vi "Get cif_manager_PluginInfo.vi"(8 "error in (no error)":errorcluster, 11 "gRPCid":T1) -> (0 "error out":errorcluster, 2 "package_templatemessage":T2, 3 "gRPCid out":T1)   [LabVIEW 2021, in "CIF_Launcher_server.lvlib"]
uses:
  CIF_Launcher_server.lvlib
  cif_manager_PluginInfo.ctl
  cif_common_ShortVersion.ctl
  cif_plugincore_StatusData.ctl
  cif_plugincore_StatusData_PluginState.ctl
  cif_plugincore_TimingStatistics.ctl
  cif_common_TimingStats.ctl
  cif_plugincore_FifoStatistics.ctl
  cif_plugincore_Error.ctl
  cif_plugincore_MonitorDoubles.ctl
  cif_plugincore_MonitorU64.ctl
  cif_plugincore_MonitorI64.ctl
  <vilib>/gRPC/LabVIEW gRPC Library/Shared/grpcId.ctl
  cif_manager_PluginInfo_Flat.ctl
  cif_common_ShortVersion_Flat.ctl
  cif_plugincore_StatusData_Flat.ctl
  cif_plugincore_TimingStatistics_Flat.ctl
  cif_common_TimingStats_Flat.ctl
  cif_plugincore_FifoStatistics_Flat.ctl
  cif_plugincore_Error_Flat.ctl
  cif_plugincore_MonitorDoubles_Flat.ctl
  cif_plugincore_MonitorU64_Flat.ctl
  cif_plugincore_MonitorI64_Flat.ctl
  2ed25e12-861d-4677-8ead-ace2906b2041.vi
  <vilib>/gRPC/LabVIEW gRPC Library/Shared/TranslateGrpcError.vi
  FlatToRichcif_common_ShortVersion.vi
  FlatToRichcif_plugincore_StatusData.vi
  FlatToRichcif_plugincore_TimingStatistics.vi
  FlatToRichcif_plugincore_FifoStatistics.vi
  FlatToRichcif_plugincore_Error.vi
  FlatToRichcif_plugincore_MonitorDoubles.vi
  FlatToRichcif_plugincore_MonitorU64.vi
  FlatToRichcif_plugincore_MonitorI64.vi
  FlatToRichcif_common_TimingStats.vi
  <vilib>/gRPC/LabVIEW gRPC Library/Server API/Server/Get Server DLL Path.vi
  <vilib>/Utility/error.llb/Error Cluster From Error Code.vi
  <vilib>/gRPC/LabVIEW gRPC Library/grpc-lvsupport-release.lvlib
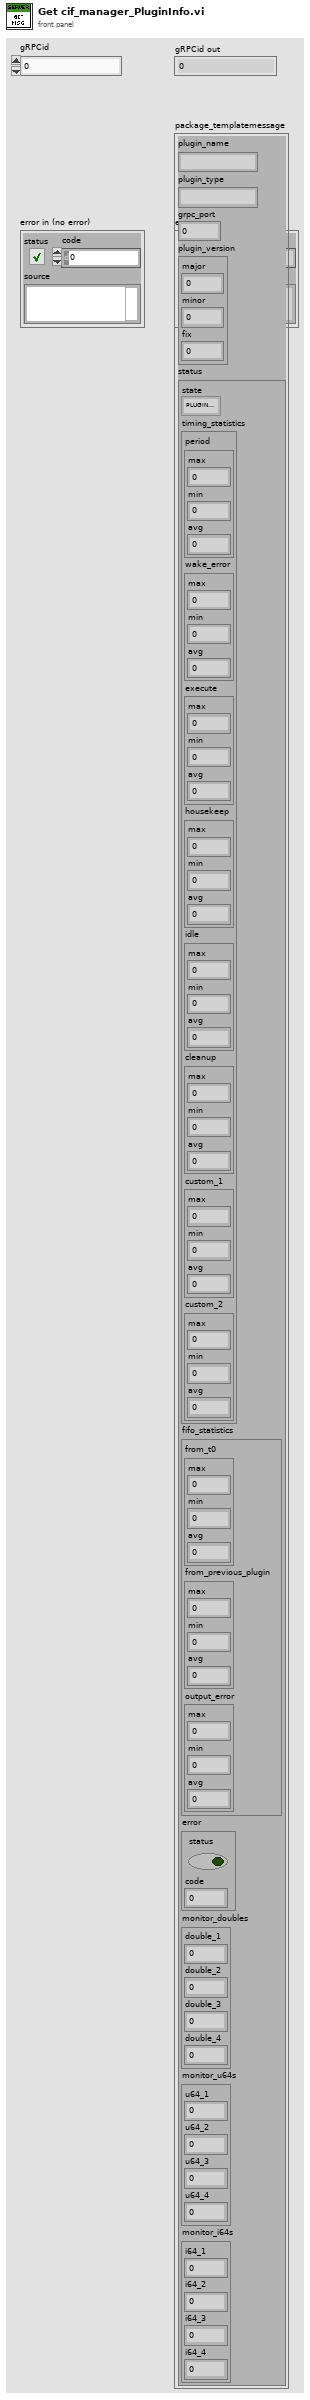
[diagram p1: front panel]
types:
  T1 = typedef "grpc-lvsupport-release.lvlib/grpcId.ctl" = u64
  T2 = typedef "CIF_Launcher_server.lvlib/cif_manager_PluginInfo.ctl" = cluster{"plugin_name":string, "plugin_type":string, "grpc_port":i32, "plugin_version":T3, "status":T4}
  T3 = typedef "CIF_Launcher_server.lvlib/cif_common_ShortVersion.ctl" = cluster{"major":u32, "minor":u32, "fix":u32}
  T4 = typedef "CIF_Launcher_server.lvlib/cif_plugincore_StatusData.ctl" = cluster{"state":T5, "timing_statistics":T6, "fifo_statistics":T8, "error":T9, "monitor_doubles":T10, "monitor_u64s":T11, "monitor_i64s":T12}
  T5 = typedef "CIF_Launcher_server.lvlib/cif_plugincore_StatusData_PluginState.ctl" = enum32{"PLUGINSTATE_UNKNOWN", "PLUGINSTATE_CREATING", "PLUGINSTATE_LISTENING", "PLUGINSTATE_RUNNING", "PLUGINSTATE_CLEANINGUP", "PLUGINSTATE_DESTROYING"}
  T6 = typedef "CIF_Launcher_server.lvlib/cif_plugincore_TimingStatistics.ctl" = cluster{"period":T7, "wake_error":T7, "execute":T7, "housekeep":T7, "idle":T7, "cleanup":T7, "custom_1":T7, "custom_2":T7}
  T7 = typedef "CIF_Launcher_server.lvlib/cif_common_TimingStats.ctl" = cluster{"max":i64, "min":i64, "avg":dbl}
  T8 = typedef "CIF_Launcher_server.lvlib/cif_plugincore_FifoStatistics.ctl" = cluster{"from_t0":T7, "from_previous_plugin":T7, "output_error":T7}
  T9 = typedef "CIF_Launcher_server.lvlib/cif_plugincore_Error.ctl" = cluster{"status":bool, "code":i32}
  T10 = typedef "CIF_Launcher_server.lvlib/cif_plugincore_MonitorDoubles.ctl" = cluster{"double_1":dbl, "double_2":dbl, "double_3":dbl, "double_4":dbl}
  T11 = typedef "CIF_Launcher_server.lvlib/cif_plugincore_MonitorU64.ctl" = cluster{"u64_1":u64, "u64_2":u64, "u64_3":u64, "u64_4":u64}
  T12 = typedef "CIF_Launcher_server.lvlib/cif_plugincore_MonitorI64.ctl" = cluster{"i64_1":i64, "i64_2":i64, "i64_3":i64, "i64_4":i64}
  T13 = typedef "CIF_Launcher_server.lvlib/cif_manager_PluginInfo_Flat.ctl" = cluster{"plugin_name":string, "plugin_type":string, "grpc_port":i32, "plugin_version":T14, "status":T15}
  T14 = typedef "CIF_Launcher_server.lvlib/cif_common_ShortVersion_Flat.ctl" = cluster{"major":u32, "minor":u32, "fix":u32}
  T15 = typedef "CIF_Launcher_server.lvlib/cif_plugincore_StatusData_Flat.ctl" = cluster{"state":T5, "timing_statistics":T16, "fifo_statistics":T18, "error":T19, "monitor_doubles":T20, "monitor_u64s":T21, "monitor_i64s":T22}
  T16 = typedef "CIF_Launcher_server.lvlib/cif_plugincore_TimingStatistics_Flat.ctl" = cluster{"period":T17, "wake_error":T17, "execute":T17, "housekeep":T17, "idle":T17, "cleanup":T17, "custom_1":T17, "custom_2":T17}
  T17 = typedef "CIF_Launcher_server.lvlib/cif_common_TimingStats_Flat.ctl" = cluster{"max":i64, "min":i64, "avg":dbl}
  T18 = typedef "CIF_Launcher_server.lvlib/cif_plugincore_FifoStatistics_Flat.ctl" = cluster{"from_t0":T17, "from_previous_plugin":T17, "output_error":T17}
  T19 = typedef "CIF_Launcher_server.lvlib/cif_plugincore_Error_Flat.ctl" = cluster{"status":bool, "code":i32}
  T20 = typedef "CIF_Launcher_server.lvlib/cif_plugincore_MonitorDoubles_Flat.ctl" = cluster{"double_1":dbl, "double_2":dbl, "double_3":dbl, "double_4":dbl}
  T21 = typedef "CIF_Launcher_server.lvlib/cif_plugincore_MonitorU64_Flat.ctl" = cluster{"u64_1":u64, "u64_2":u64, "u64_3":u64, "u64_4":u64}
  T22 = typedef "CIF_Launcher_server.lvlib/cif_plugincore_MonitorI64_Flat.ctl" = cluster{"i64_1":i64, "i64_2":i64, "i64_3":i64, "i64_4":i64}
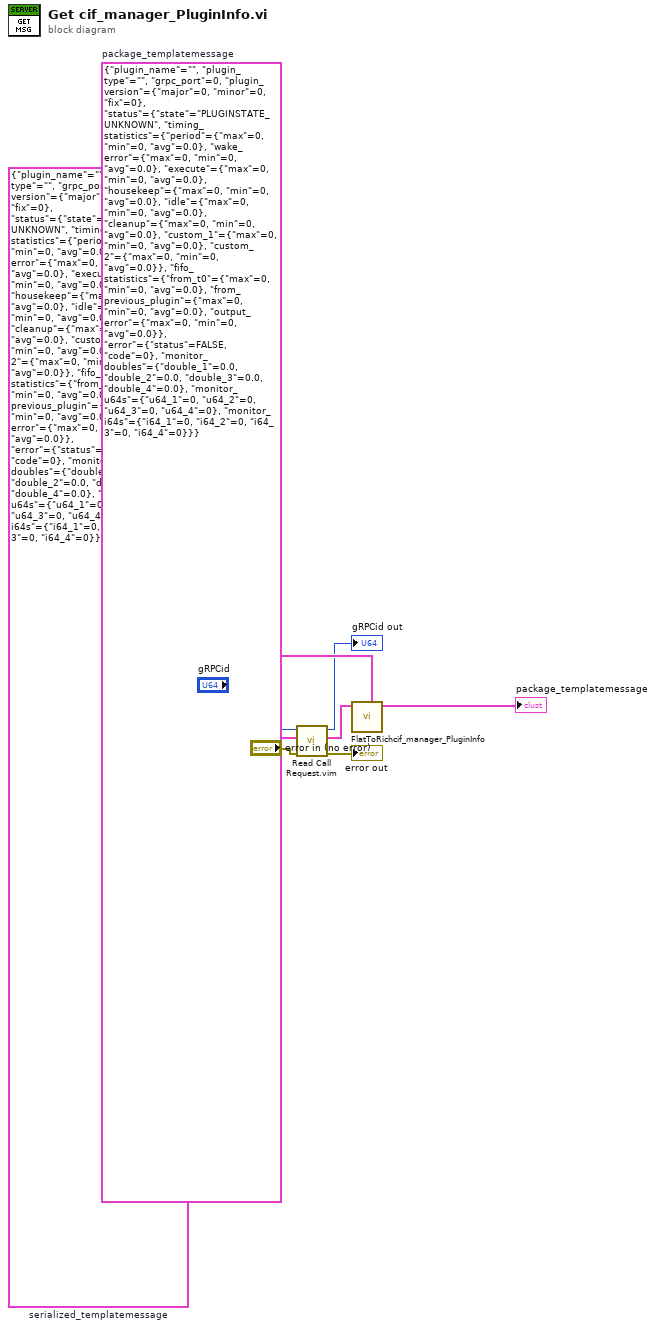
[diagram p0: block diagram]
diagram:
  w6 = T13 {"plugin_name"="", "plugin_type"="", "grpc_port"=0, "plugin_version"={"major"=0, "minor"=0, "fix"=0}, "status"={"state"=enum."PLUGINSTATE_UNKNOWN", "timing_statistics"={"period"={"max"=0, "min"=0, "avg"=0.0}, "wake_error"={"max"=0, "min"=0, "avg"=0.0}, "execute"={"max"=0, "min"=0, "avg"=0.0}, "housekeep"={"max"=0, "min"=0, "avg"=0.0}, "idle"={"max"=0, "min"=0, "avg"=0.0}, "cleanup"={"max"=0, "min"=0, "avg"=0.0}, "custom_1"={"max"=0, "min"=0, "avg"=0.0}, "custom_2"={"max"=0, "min"=0, "avg"=0.0}}, "fifo_statistics"={"from_t0"={"max"=0, "min"=0, "avg"=0.0}, "from_previous_plugin"={"max"=0, "min"=0, "avg"=0.0}, "output_error"={"max"=0, "min"=0, "avg"=0.0}}, "error"={"status"=FALSE, "code"=0}, "monitor_doubles"={"double_1"=0.0, "double_2"=0.0, "double_3"=0.0, "double_4"=0.0}, "monitor_u64s"={"u64_1"=0, "u64_2"=0, "u64_3"=0, "u64_4"=0}, "monitor_i64s"={"i64_1"=0, "i64_2"=0, "i64_3"=0, "i64_4"=0}}}  # serialized_templatemessage
  w5 = T2 {"plugin_name"="", "plugin_type"="", "grpc_port"=0, "plugin_version"={"major"=0, "minor"=0, "fix"=0}, "status"={"state"=enum."PLUGINSTATE_UNKNOWN", "timing_statistics"={"period"={"max"=0, "min"=0, "avg"=0.0}, "wake_error"={"max"=0, "min"=0, "avg"=0.0}, "execute"={"max"=0, "min"=0, "avg"=0.0}, "housekeep"={"max"=0, "min"=0, "avg"=0.0}, "idle"={"max"=0, "min"=0, "avg"=0.0}, "cleanup"={"max"=0, "min"=0, "avg"=0.0}, "custom_1"={"max"=0, "min"=0, "avg"=0.0}, "custom_2"={"max"=0, "min"=0, "avg"=0.0}}, "fifo_statistics"={"from_t0"={"max"=0, "min"=0, "avg"=0.0}, "from_previous_plugin"={"max"=0, "min"=0, "avg"=0.0}, "output_error"={"max"=0, "min"=0, "avg"=0.0}}, "error"={"status"=FALSE, "code"=0}, "monitor_doubles"={"double_1"=0.0, "double_2"=0.0, "double_3"=0.0, "double_4"=0.0}, "monitor_u64s"={"u64_1"=0, "u64_2"=0, "u64_3"=0, "u64_4"=0}, "monitor_i64s"={"i64_1"=0, "i64_2"=0, "i64_3"=0, "i64_4"=0}}}  # package_templatemessage
  n1 = call "Read Call Request.vim"("error in"="error in (no error)", "Request Type"=w6, "gRPCid in"="gRPCid") -> ("error out"=→"error out":errorcluster, "Request Data"=w4:T13, "gRPCid out"=→"gRPCid out":T1)  [unwired: 6 in]
  n2 = call "FlatToRichcif_manager_PluginInfo.vi"("OutputClusterType"=w5, "InputCluster"=w4) -> ("OutputCluster"=→"package_templatemessage":T2)  [unwired: 9 in]
